vi "Framework.Rx.Begin.vi"(8 "error in (no error)":errorcluster, 11 "Framework in":refnum<class "Framework.lvclass">) -> (0 "error out":errorcluster, 3 "Framework out":refnum<class "Framework.lvclass">)   [LabVIEW 2017, in "DSF Core.lvlib" / "Framework.lvclass"]
uses:
  Framework.lvclass
  Framework.lvclass/Framework.ctl
  Status/Framework Status.lvclass/Framework Status.ctl
  Status/Framework Performance.lvclass/Framework Performance.ctl
  Status/Framework Status.lvclass
  Status/Framework Performance.lvclass
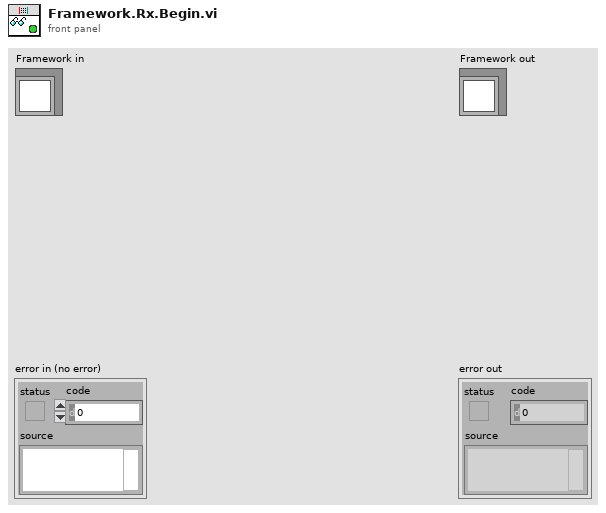
[diagram p1: front panel]
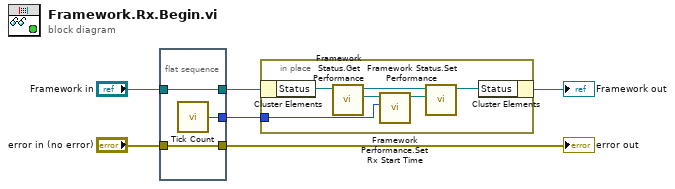
[diagram p0: block diagram]
diagram:
  n1 = flat-sequence {
    tunnel: "Framework in" -> [w8]
    tunnel: "error in (no error)" -> [w9]
    tunnel: [w9] -> w4
    tunnel: [w8] -> w3
    tunnel: [w7] -> w2
    frame #0 {
      n2 = call "Tick Count"() -> ("Tick Count(uSec)"=w7:u32)
    }
  }
  n3 = in-place {
    in-place-border: w2 -> [w10]
    n4 = in-place-cluster #1(w3) -> ("Status"=w15:refnum<class "Framework Status.lvclass">)
    n5 = call "Framework Status.Get Performance.vi"("Framework Status in"=w15) -> ("Framework Performance"=w14:refnum<class "Framework Performance.lvclass">, "Framework Status out"=w13:refnum<class "Framework Status.lvclass">)  [unwired: 9 in]
    n6 = call "Framework Performance.Set Rx Start Time.vi"("Rx start time"=w10, "Framework Performance in"=w14) -> ("Framework Performance out"=w12:refnum<class "Framework Performance.lvclass">)  [unwired: 9 in]
    n7 = call "Framework Status.Set Performance.vi"("Framework Performance"=w12, "Framework Status in"=w13) -> ("Framework Status out"=w11:refnum<class "Framework Status.lvclass">)  [unwired: 9 in]
    n8 = in-place-cluster #1("Status"=w11) -> (→"Framework out":refnum<class "Framework.lvclass">)
  }
  "error out" <- w4
